vi "FGV Background-Daten.vi"(0 "Background Daten":cluster{"Ramp Pattern":dbl[], dbl[]}[](array[cluster]), 5 "Background aktiv":bool, 11 "error in (no error)":errorcluster caption="Fehler (Eingang, kein Fehler)", 12 "Aktion":T1) -> (1 "Zeitstempel GB":timestamp, 3 "Zeitstempel":timestamp, 4 "Background Daten":cluster{"Ramp Pattern":dbl[], dbl[]}[](array[cluster]), 6 "Background aktiv":bool, 8 "Referenz-200":cluster{"Ramp Pattern":dbl[], dbl[]}, 10 "Referenz":cluster{"Ramp Pattern":dbl[], dbl[]}, 14 "Golden Background":cluster{dbl[], "[Y]":sgl[]}, 15 "error out":errorcluster caption="Fehler (Ausgang)")   [LabVIEW 2020, in "FT-IR.lvlib" / "Get Spectra.lvlib"]
uses:
  Get Spectra.lvlib
  Aktion FGV Background-Daten.ctl
  ReadLabFile/Spectrum FILE.ctl
  ReadLabFile/User arrays.ctl
  ReadLabFile/Sub spectra.ctl
  ReadLabFile/Spectrum.ctl
  Allgemein/allgemeine Sub-VIs.lvlib
  ReadLabFile/Read Lab File.lvlib
panel:
  in  "Spectrum  FILE Name":path=path "D:/IAG_Data/Communication/GoldenBackground/backgrnd.lab"
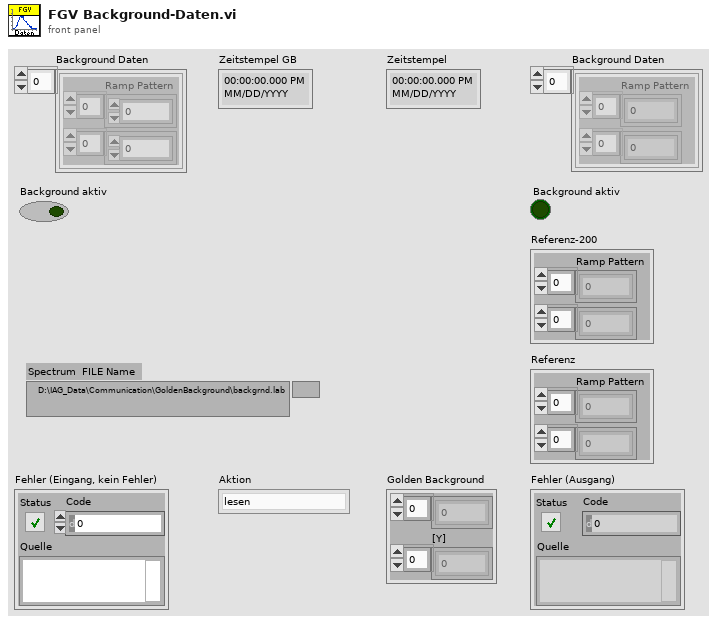
[diagram p1: front panel]
types:
  T1 = typedef "FT-IR.lvlib/Get Spectra.lvlib/Aktion FGV Background-Daten.ctl" = enum16{"lesen", "schreiben", "Background aktiv", "Referenz", "laden", "speichern", "Plot sichtbar"}
  T2 = typedef "FT-IR.lvlib/Read Lab File.lvlib/Spectrum FILE.ctl" = cluster{"MEMO":string, "User arrays":T3, "SPECTRA":T4}
  T3 = typedef "FT-IR.lvlib/Read Lab File.lvlib/User arrays.ctl" = cluster{"Tag":string, "User double":dbl[]}[]
  T4 = typedef "FT-IR.lvlib/Read Lab File.lvlib/Sub spectra.ctl" = cluster{"Tag":string, "DATE AND TIME":u32, "spectrum":T5}[]
  T5 = typedef "FT-IR.lvlib/Read Lab File.lvlib/Spectrum.ctl" = cluster{"x0":dbl, "dx":dbl, "[Y]":sgl[]}
  T6 = cluster{cluster{"Ramp Pattern":dbl[], dbl[]}, "seconds since 1Jan1904":timestamp}
  T7 = cluster{"Tag":string, "DATE AND TIME":u32, "spectrum":T5}
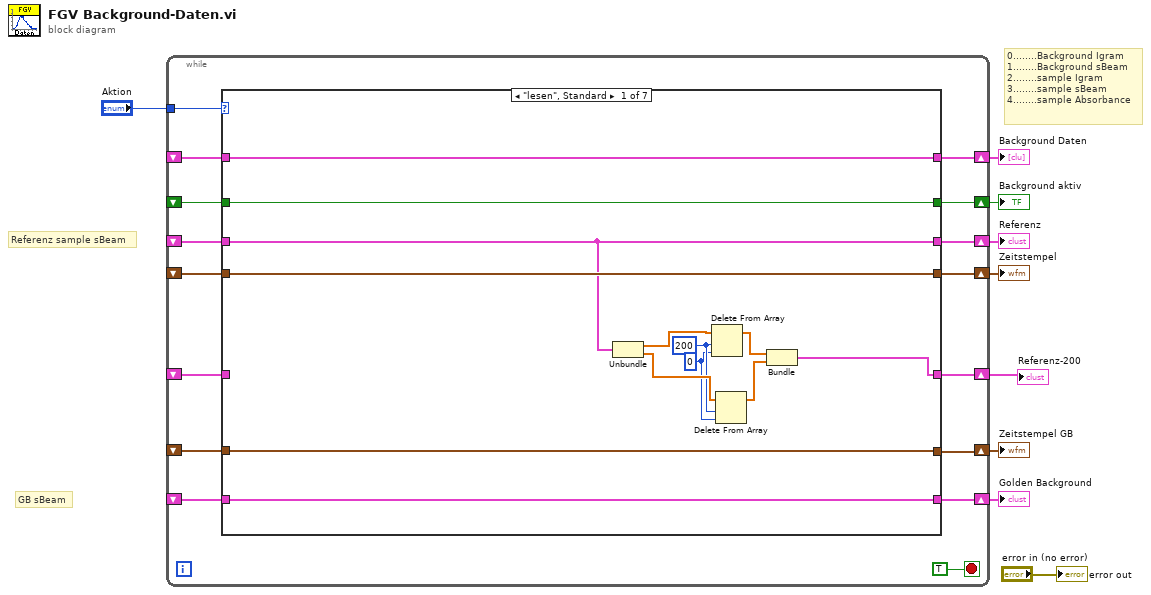
[diagram p0: block diagram]
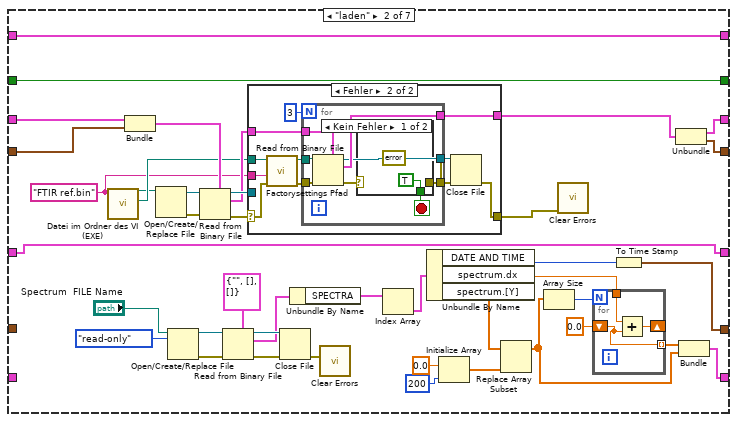
[diagram p2: hidden frame]
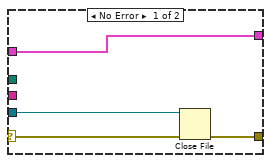
[diagram p3: hidden frame]
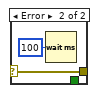
[diagram p4: hidden frame]
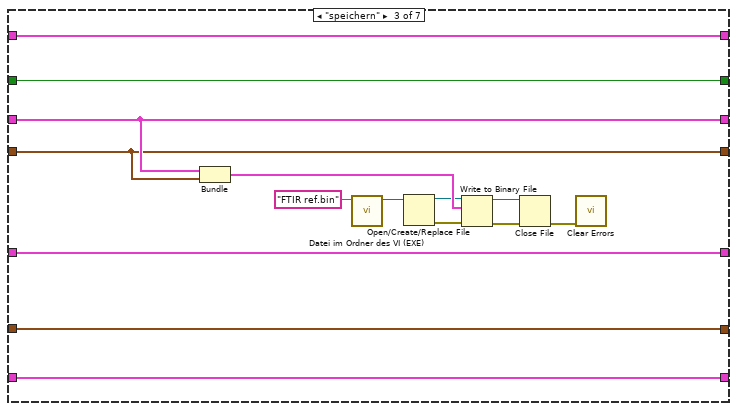
[diagram p5: hidden frame]
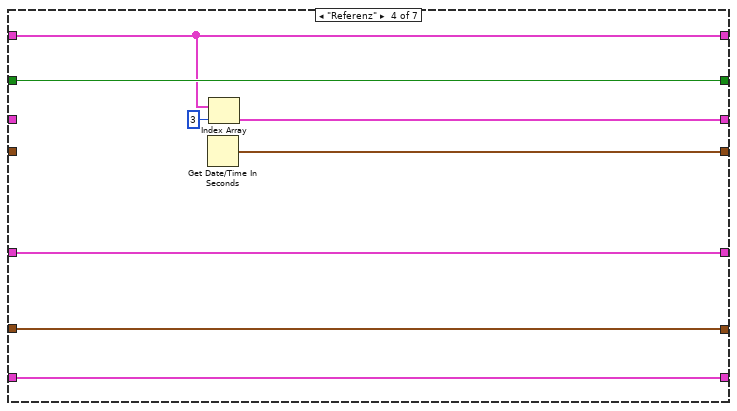
[diagram p6: hidden frame]
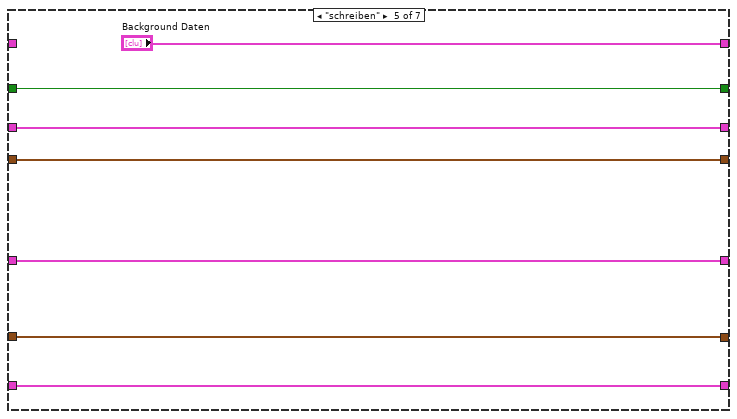
[diagram p7: hidden frame]
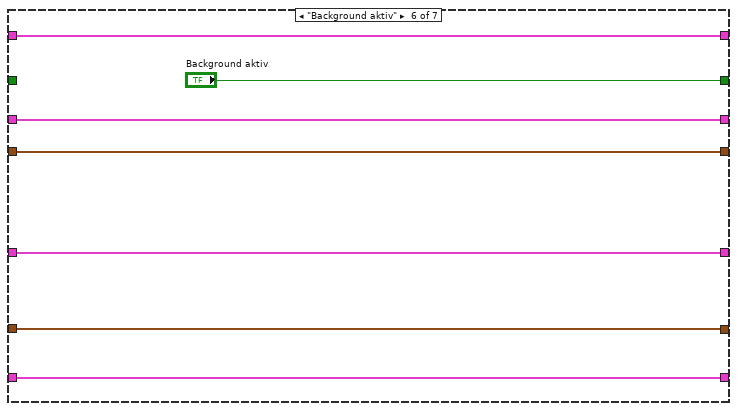
[diagram p8: hidden frame]
diagram:
  # "GB sBeam"
  # "Referenz sample sBeam"
  # "0........Background Igram\n1........Background sBeam\n2........sample Igram\n3........sample sBeam\n4........sample Absorbance"
  n1 = while {
    tunnel: "Aktion" -> [w24]
    shift-right: [w23] -> w8
    shift-left: _ -> [w22]
    shift-right: [w21] -> w7
    shift-left: _ -> [w20]
    shift-right: [w19] -> w6
    shift-left: _ -> [w18]
    shift-right: [w17] -> w5
    shift-left: _ -> [w16]
    shift-right: [w15] -> w3
    shift-left: _ -> [w14]
    shift-right: [w13] -> w2
    shift-left: _ -> [w12]
    shift-right: [w11] -> w1
    shift-left: _ -> [w10]
    stop <- TRUE stop-if-true
    n2 = case shown="\"lesen\", Standard" w24 {
      tunnel: [w38 w79 w124 w131 "Background Daten" w146 w149] -> w23
      tunnel: w22 -> [w38 w79 w124 w131 _ w146 w149]
      tunnel: [w37 w78 w123 w132 w138 "Background aktiv" w150] -> w21
      tunnel: w20 -> [w37 w78 w123 w132 w138 _ w150]
      tunnel: [w29 w74 w121 w126 w137 w144 w151] -> w19
      tunnel: w18 -> [w29 w76 w121 _ w137 w144 w151]
      tunnel: [w36 w73 w120 w129 w136 w143 w152] -> w17
      tunnel: w16 -> [w36 w75 w120 _ w136 w143 w152]
      tunnel: [w35 w43 w112 w128 w135 w142 w153] -> w15
      tunnel: w14 -> [w35 _ w112 w128 w135 w142 w153]
      tunnel: [w34 w41 w111 w127 w134 w141 w148] -> w13
      tunnel: w12 -> [w34 _ w111 w127 w134 w141 w148]
      tunnel: [w28 w39 w110 w125 w133 w140 w147] -> w11
      tunnel: w10 -> [_ w39 w110 w125 w133 w140 w147]
      frame "lesen", Default {
        w30 = 0 ("Länge")
        w31 = 200 ("Index")
        n3 = Unbundle(w29) -> ("Ramp Pattern"=w33:dbl[], w32:dbl[])
        n4 = Delete From Array(array=w33, length=w31, index=w30) -> (array with subset deleted=w27:dbl[])  [unwired: 1 out]
        n5 = Delete From Array(array=w32, length=w31, index=w30) -> (array with subset deleted=w26:dbl[])  [unwired: 1 out]
        n6 = Bundle("Ramp Pattern"=w27, w26) -> (w28:cluster{"Ramp Pattern":dbl[], dbl[]})  [unwired: 1 in]
      }
      frame "laden" {
        w67 = "FTIR ref.bin" ("Dateiname")
        n7 = call "Datei im Ordner des VI (EXE).vi"("Dateiname"=w67) -> ("Ordner des Haupt-VIs"=w68:path, "Dateipfad im Ordner des Haupt-VIs"=w65:path)  [unwired: 8 in, 1 out]
        n8 = Bundle(w76, "seconds since 1Jan1904"=w75) -> (w77:T6)  [unwired: 1 in]
        n9 = Open/Create/Replace File(file path (use dialog)=w65) -> (refnum out=w64:refnum<file>, error out=w66:errorcluster)  [unwired: 5 in, 1 out]
        n10 = Open/Create/Replace File(file path (use dialog)="Spectrum  FILE Name", access (0:read/write)=enum16{"read/write", "read-only", "write-only"}."read-only" ("Zugriff (0:Lesen/Schreiben)")) -> (refnum out=w63:refnum<file>, error out=w62:errorcluster)  [unwired: 1 in, 4 out]
        n11 = Read from Binary File(5:w77, 8:w66, 11:w64) -> (0:w72:errorcluster, 2:w69:T6, 3:w71:refnum<file>)  [unwired: 3 in, 1 out]
        n12 = Read from Binary File(5:T2 {"MEMO"="", "User arrays"=[], "SPECTRA"=[]} ("empty Spectrum FILE"), 8:w62, 11:w63) -> (0:w58:errorcluster, 2:w53:T2, 3:w61:refnum<file>)  [unwired: 4 out]
        n13 = case shown="Fehler" w72 {
          selector: w72 -> [w85 w89]
          tunnel: w68 -> [_ w90]
          tunnel: w69 -> [w86 w88]
          tunnel: [w86 w96] -> w40
          tunnel: [w83 w94] -> w70
          tunnel: w71 -> [w84 _]
          tunnel: w67 -> [_ w87]
          frame No Error {
            n14 = Close File(refnum=w84, error in=w85) -> (error out=w83:errorcluster)  [unwired: 1 out]
          }
          frame Error {
            n15 = call "Factorysettings Pfad.vi"("error in (no error)"=w89, "Dateiname"=w87, "Ordner des Haupt-VIs"=w90) -> ("error out"=w91:errorcluster, "Pfad Factorysettings"=w92:path)  [unwired: 7 in]
            n16 = for {
              N: 3 -> [_]
              tunnel: w91 -> [w103]
              tunnel: w92 -> [w102]
              tunnel: [w101] -> w96
              tunnel: [w100] -> w95
              tunnel: [w99] -> w93
              tunnel: w88 -> [w98]
              stop <- w104 stop-if-true
              n17 = Read from Binary File(5:w98, 8:w103, 11:w102) -> (0:w105:errorcluster, 2:w101:T6, 3:w99:refnum<file>)  [unwired: 3 in, 1 out]
              n18 = case shown="Kein Fehler" w105 {
                selector: w105 -> [_ w108]
                tunnel: [TRUE _] -> w104
                tunnel: [errorcluster {"status"=FALSE, "code"=0, "source"=""} ("error IO") w108] -> w100
                frame No Error {
                }
                frame Error {
                  n19 = Wait (ms)(milliseconds to wait=u32 100 ("Zu wartende ms")) -> ()  [unwired: 1 out]
                }
              }
            }
            n20 = Close File(refnum=w93, error in=w95) -> (error out=w94:errorcluster)  [unwired: 1 out]
          }
        }
        n21 = Close File(refnum=w61, error in=w58) -> (error out=w56:errorcluster)  [unwired: 1 out]
        n22 = Unbundle By Name(w53) -> ("SPECTRA"=w50:T4)
        n23 = call <vilib>:"Clear Errors.vi"("error in (no error)"=w56) -> ()  [unwired: 5 in, 2 out]
        n24 = Index Array(array=w50) -> (element=w49:T7)  [unwired: 1 in]
        n25 = Unbundle By Name(w49) -> ("DATE AND TIME"=w42:u32, "spectrum.dx"=w46:dbl, "spectrum.[Y]"=w48:sgl[])
        n26 = Initialize Array(0.0 ("Element"), 200 ("Dimensionsgröße")) -> (w47:dbl[])
        n27 = Replace Array Subset(array=w48, new element=w47) -> (w44:sgl[])  [unwired: 1 in]
        n28 = Array Size(array=w44) -> (size(s)=w55:i32)
        n29 = call <vilib>:"Clear Errors.vi"("error in (no error)"=w70) -> ()  [unwired: 5 in, 2 out]
        n30 = for {
          N: w55 -> [_]
          tunnel: [w81] -> w45 mode=indexing
          shift-right: [w82] -> _
          shift-left: 0.0 -> [w81]
          tunnel: w46 -> [w80]
          n31 = Add(x=w80, y=w81) -> (x+y=w82:dbl)
        }
        n32 = To Time Stamp(1:w42) -> (0:w41:timestamp)
        n33 = Unbundle(w40) -> (w74:cluster{"Ramp Pattern":dbl[], dbl[]}, "seconds since 1Jan1904"=w73:timestamp)
        n34 = Bundle(w45, "[Y]"=w44) -> (w43:cluster{dbl[], "[Y]":sgl[]})  [unwired: 1 in]
      }
      frame "speichern" {
        n35 = Bundle(w121, "seconds since 1Jan1904"=w120) -> (w119:T6)  [unwired: 1 in]
        n36 = call "Datei im Ordner des VI (EXE).vi"("Dateiname"="FTIR ref.bin") -> ("Dateipfad im Ordner des Haupt-VIs"=w118:path)  [unwired: 8 in, 2 out]
        n37 = Open/Create/Replace File(file path (use dialog)=w118) -> (refnum out=w117:refnum<file>, error out=w113:errorcluster)  [unwired: 5 in, 1 out]
        n38 = Write to Binary File(file (use dialog)=w117, data=w119, error in=w113) -> (refnum out=w115:refnum<file>, error out=w116:errorcluster)  [unwired: 3 in, 1 out]
        n39 = Close File(refnum=w115, error in=w116) -> (error out=w114:errorcluster)  [unwired: 1 out]
        n40 = call <vilib>:"Clear Errors.vi"("error in (no error)"=w114) -> ()  [unwired: 5 in, 2 out]
      }
      frame "Referenz" {
        n41 = Get Date/Time In Seconds() -> (seconds since 1Jan1904=w129:timestamp)
        n42 = Index Array(array=w131, index=3 ("Index")) -> (element=w126:cluster{"Ramp Pattern":dbl[], dbl[]})
      }
      frame "schreiben" {
      }
      frame "Background aktiv" {
      }
      frame "Plot sichtbar" {
      }
    }
  }
  "Background Daten" <- w8
  "Background aktiv" <- w7
  "Referenz" <- w6
  "Zeitstempel" <- w5
  "Golden Background" <- w3
  "Zeitstempel GB" <- w2
  "Referenz-200" <- w1
  "error out" <- "error in (no error)"
